vi "gRPC_Wrapper_VISA_implement_v1.0.0.vi"() -> ()   [LabVIEW 2022 SP3]
uses:
  <vilib>/Instr/_visa.llb/VISA Open Access Mode.ctl
panel:
  in  "Refresh":bool
  in  "VISA CLOSE":bool
  in  "VISA resource name":refnum<visa-resource-name>="test_LabVIEW"
  out "Waveform Graph":dbl[](graph)
  out "Waveform Chart":dbl(graph)
  out "Gain":string
  in  "Select Command":string(combo)
  out "Active":bool
  in  "Send":bool
  in  "Type Command":string
  in  "Query":bool
  out "Command":string
  out "Dot-Notation Address":string
  out "Computer Hostname":string
  out "Resource Manufacturer Name":string
  out "Resource Manufacturer Identification":u16
  out "Version of Specification":u32
  out "Resource Lock State":u32(ring) items=["Unlocked", "Exclusive", "Shared"]
  out "Resource Name":string
  out "Read return count":u32
  out "Write return count":u32
  out "Respose From Device":string
  # "Operations"
  # "Informations"
  # "Device Signal Parameters"
  # "Graph / Chart"
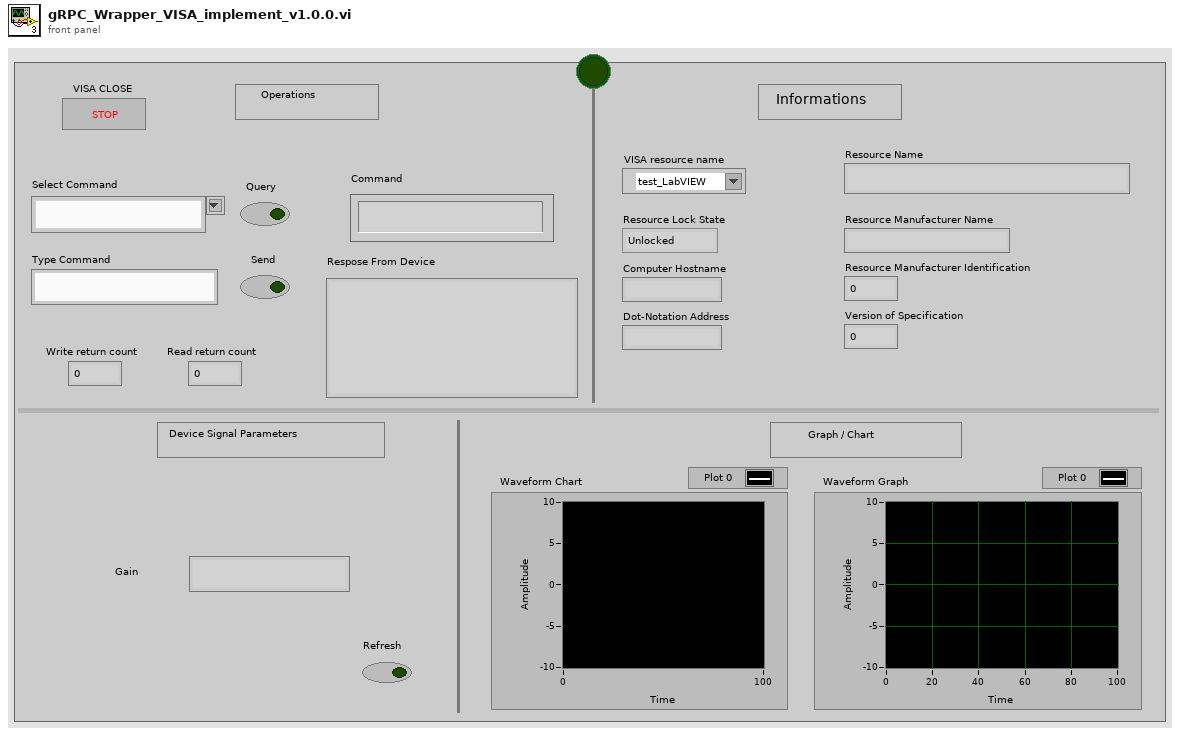
[diagram p1: front panel]
types:
  T1 = typedef "VISA Open Access Mode.ctl" = u32
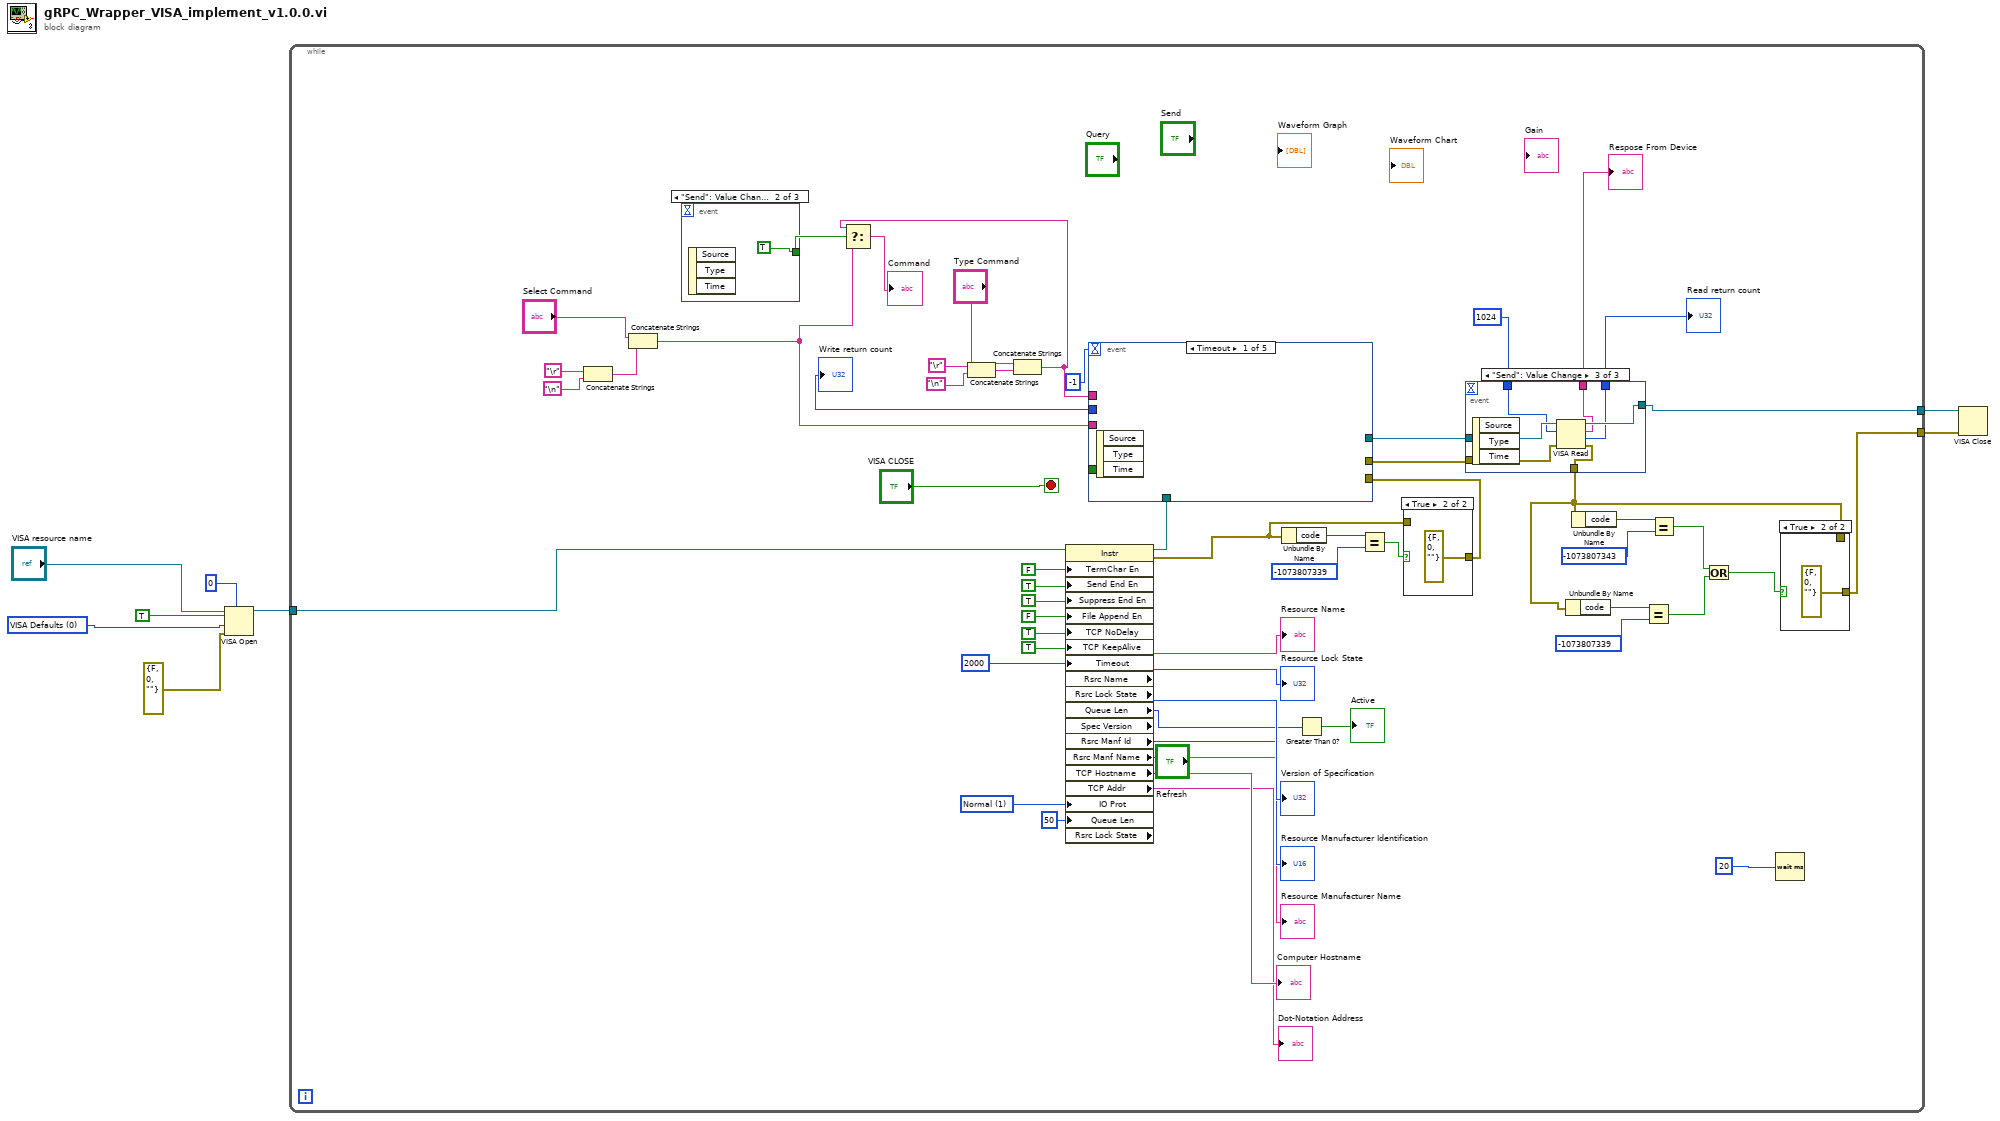
[diagram p0: block diagram]
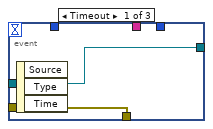
[diagram p2: hidden frame]
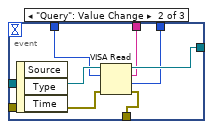
[diagram p3: hidden frame]
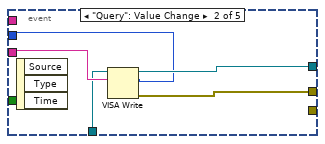
[diagram p6: hidden frame]
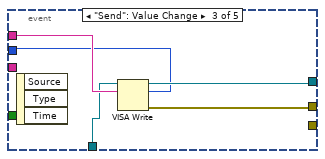
[diagram p7: hidden frame]
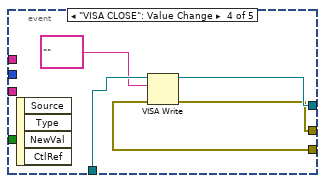
[diagram p8: hidden frame]
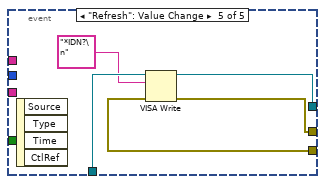
[diagram p9: hidden frame]
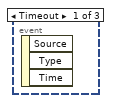
[diagram p10: hidden frame]
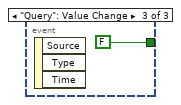
[diagram p11: hidden frame]
diagram:
  w3 = T1 0 items=["VISA Defaults"=0, "Exclusive Lock"=1, "Load Configured Settings"=4] ("Access Mode")
  n1 = VISA Open(timeout (0)=u32 0 ("VISA Open timeout (0)"), duplicate session (F)=TRUE, access mode=w3, error in (no error)=errorcluster {"status"=FALSE, "code"=0, "source"=""}, VISA resource name="VISA resource name") -> (VISA resource name=w1:refnum<visa-resource-name>)  [unwired: 1 out]
  n2 = while {
    tunnel: [w11] -> w8
    tunnel: [w10] -> w7
    tunnel: w1 -> [w9]
    stop <- "VISA CLOSE" stop-if-true
    w50 = u16 1 items=["Normal"=1, "VXI/FDC"=2, "GPIB/HS488"=3, "Serial-TCPIP-USB/488 Strings"=4, "USBTMC/Vendor-Specific"=5] ("Message Based Settings:IO Protocol")
    n3 = Concatenate Strings("\r", "\n") -> (w36:string)
    n4 = Concatenate Strings("Select Command", w36) -> (w32:string)
    n5 = event shown="[1] \"Send\": Value Change" {
      selector: _ -> [_ _ _]
      dyn-events: _ -> [_ _ _]
      timeout: _ -> [_ _ _]
      tunnel: [_ TRUE FALSE] -> w38
      event Timeout {
        n6 = event-data() -> ()  [unwired: 1 in, 3 out]
      }
      event "Send": Value Change {
        n7 = event-data() -> ()  [unwired: 1 in, 3 out]
      }
      event "Query": Value Change {
        n8 = event-data() -> ()  [unwired: 1 in, 3 out]
      }
    }
    n9 = Concatenate Strings("\r", "\n") -> (w37:string)
    n10 = Concatenate Strings("Type Command", w37) -> (w31:string)
    n11 = Select(t=w31, s=w38, f=w32) -> (s? t:f=→"Command":string)
    n12 = property class="Instr" props=["TermChar En", "Send End En", "Suppress End En", "File Append En", "TCP NoDelay", "TCP KeepAlive", "Timeout", "Rsrc Name", "Rsrc Lock State", "Queue Len", "Spec Version", "Rsrc Manf Id", "Rsrc Manf Name", "TCP Hostname", "TCP Addr", "IO Prot", "Queue Len", "Rsrc Lock State"](reference=w9, "TermChar En"=FALSE ("Message Based Settings:Termination Character Enable"), "Send End En"=TRUE ("Message Based Settings:Send End Enable"), "Suppress End En"=TRUE ("Message Based Settings:Suppress End Enable"), "File Append En"=FALSE ("Message Based Settings:File Append Enable"), "TCP NoDelay"=TRUE ("TCP/IP Settings:No Packet Delay"), "TCP KeepAlive"=TRUE ("TCP/IP Settings:Keep-Alive Packets"), "Timeout"=u32 2000 ("General Settings:Timeout Value"), "IO Prot"=w50, "Queue Len"=u32 50 ("General Settings:Maximum Queue Length")) -> (reference out=w30:refnum<visa-resource-name>, error out=w23:errorcluster, "Rsrc Name"=→"Resource Name":string, "Rsrc Lock State"=→"Resource Lock State":u32, "Queue Len"=w41:u32, "Spec Version"=→"Version of Specification":u32, "Rsrc Manf Id"=→"Resource Manufacturer Identification":u16, "Rsrc Manf Name"=→"Resource Manufacturer Name":string, "TCP Hostname"=→"Computer Hostname":string, "TCP Addr"=→"Dot-Notation Address":string)  [unwired: 1 in, 1 out]
    n13 = Unbundle By Name(w23) -> ("code"=w26:i32)
    n14 = Greater Than 0?(x=w41) -> (x > 0?=→"Active":bool)
    n15 = Equal?(x=w26, y=-1073807339) -> (x = y?=w25:bool)
    n16 = case shown="True" w25 {
      tunnel: [w81 errorcluster {"status"=FALSE, "code"=0, "source"=""} ("error constant")] -> w24
      tunnel: w23 -> [w81 _]
      frame False {
      }
      frame True {
      }
    }
    n17 = event shown="[0] Timeout" {
      selector: _ -> [_ _ _ _ _]
      dyn-events: _ -> [_ _ _ _ _]
      timeout: -1 -> [_ _ _ _ _]
      tunnel: [_ w89 w94 w100 w104] -> w13
      tunnel: [_ w88 w93 w99 w103] -> w12
      tunnel: [_ w86 w91 _ _] -> w46
      tunnel: w32 -> [_ w87 _ _ _]
      tunnel: w31 -> [_ _ w92 _ _]
      tunnel: w30 -> [_ w85 w90 w97 w105]
      tunnel: w24 -> [_ _ _ w98 w102]
      tunnel: [_ _ _ w95 _] -> _
      event Timeout {
        n18 = event-data() -> ()  [unwired: 1 in, 3 out]
      }
      event "Query": Value Change {
        n19 = event-data() -> ()  [unwired: 1 in, 3 out]
        n20 = VISA Write(VISA resource name=w85, write buffer=w87) -> (VISA resource name out=w89:refnum<visa-resource-name>, return count=w86:u32, error out=w88:errorcluster)  [unwired: 1 in]
      }
      event "Send": Value Change {
        n21 = event-data() -> ()  [unwired: 1 in, 3 out]
        n22 = VISA Write(VISA resource name=w90, write buffer=w92) -> (VISA resource name out=w94:refnum<visa-resource-name>, return count=w91:u32, error out=w93:errorcluster)  [unwired: 1 in]
      }
      event "VISA CLOSE": Value Change {
        n23 = event-data() -> ("NewVal"=w95:bool)  [unwired: 1 in, 3 out]
        n24 = VISA Write(VISA resource name=w97, write buffer="", error in (no error)=w98) -> (VISA resource name out=w100:refnum<visa-resource-name>, error out=w99:errorcluster)  [unwired: 1 out]
      }
      event "Refresh": Value Change {
        n25 = event-data() -> ()  [unwired: 1 in, 4 out]
        n26 = VISA Write(VISA resource name=w105, write buffer="*IDN?\n", error in (no error)=w102) -> (VISA resource name out=w104:refnum<visa-resource-name>, error out=w103:errorcluster)  [unwired: 1 out]
      }
    }
    "Write return count" <- w46
    n27 = event shown="[2] \"Send\": Value Change" {
      selector: _ -> [_ _ _]
      dyn-events: _ -> [_ _ _]
      timeout: _ -> [_ _ _]
      tunnel: u32 1024 ("byte count") -> [_ w67 w74]
      tunnel: [_ w68 w76] -> w47
      tunnel: [_ w69 w75] -> w21
      tunnel: [w65 w70 w77] -> w18
      tunnel: [w66 w71 w78] -> w10
      tunnel: w13 -> [w66 w73 w80]
      tunnel: w12 -> [w65 w72 w79]
      event Timeout {
        n28 = event-data() -> ()  [unwired: 1 in, 3 out]
      }
      event "Query": Value Change {
        n29 = event-data() -> ()  [unwired: 1 in, 3 out]
        n30 = VISA Read(VISA resource name=w73, byte count=w67, error in (no error)=w72) -> (VISA resource name out=w71:refnum<visa-resource-name>, read buffer=w69:string, return count=w68:u32, error out=w70:errorcluster)
      }
      event "Send": Value Change {
        n31 = event-data() -> ()  [unwired: 1 in, 3 out]
        n32 = VISA Read(VISA resource name=w80, byte count=w74, error in (no error)=w79) -> (VISA resource name out=w78:refnum<visa-resource-name>, read buffer=w75:string, return count=w76:u32, error out=w77:errorcluster)
      }
    }
    "Read return count" <- w47
    "Respose From Device" <- w21
    n33 = Unbundle By Name(w18) -> ("code"=w19:i32)
    n34 = Unbundle By Name(w18) -> ("code"=w29:i32)
    n35 = Equal?(x=w19, y=-1073807339) -> (x = y?=w15:bool)
    n36 = Equal?(x=w29, y=-1073807343) -> (x = y?=w16:bool)
    n37 = Or(x=w16, y=w15) -> (x .or. y?=w17:bool)
    n38 = Wait (ms)(milliseconds to wait=u32 20) -> ()  [unwired: 1 out]
    n39 = case shown="True" w17 {
      tunnel: [w83 errorcluster {"status"=FALSE, "code"=0, "source"=""} ("error constant")] -> w11
      tunnel: w18 -> [w83 _]
      frame False {
      }
      frame True {
      }
    }
  }
  n40 = VISA Close(VISA resource name=w7, error in (no error)=w8) -> ()  [unwired: 1 out]
